vi "Goniometer2.vi"() -> ()   [LabVIEW 2024]
uses:
  F:/Desktop/Goniometer_Labview/ThorLabs.MotionControl.KCube.DCServoCLI.dll
  ThorLabs.MotionControl.KCube.DCServoCLI.dll
  F:/Desktop/Goniometer_Labview/Thorlabs.MotionControl.Controls.dll
  Thorlabs.MotionControl.Controls.dll
panel:
  in  "Boolean":bool
  out "이동거리":dbl[](array[numeric])
  out "Waveform Chart":dbl[](graph)
  out "XY Graph":cluster{dbl[], dbl[]}(graph)
  out "측정값":dbl[](array[numeric])
  out "error out":errorcluster {"code" format="%.0x"}
  in  "direction":i32(ring)=2 items=["Forward"=1, "Backward"=2]
  in  "목표위치":dbl
  in  "간격":dbl
  in  "Mode":u16(ring) items=["Current", "Power"]
  out "Current":dbl
  in  "Wavelength (0.0)":dbl=1064.0
  out "Power":dbl
  in  "Serial Number":string
  in  "KCubeDCServoControl":refnum<k24>(container)
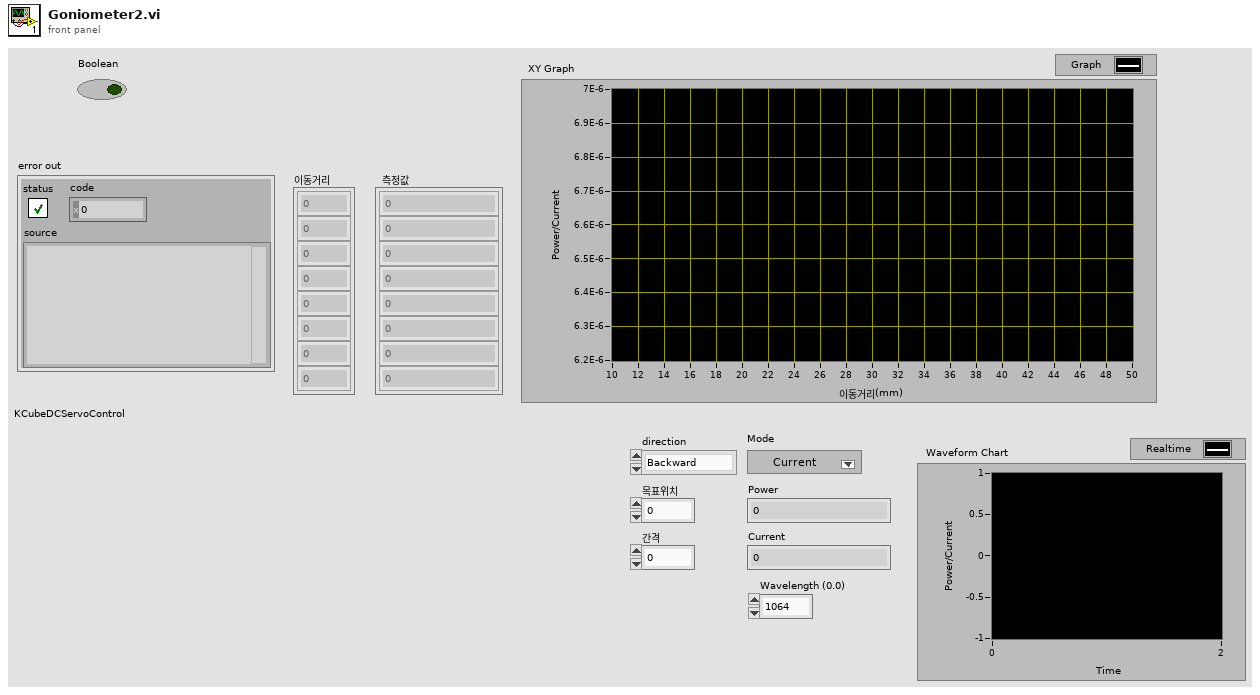
[diagram p1: front panel]
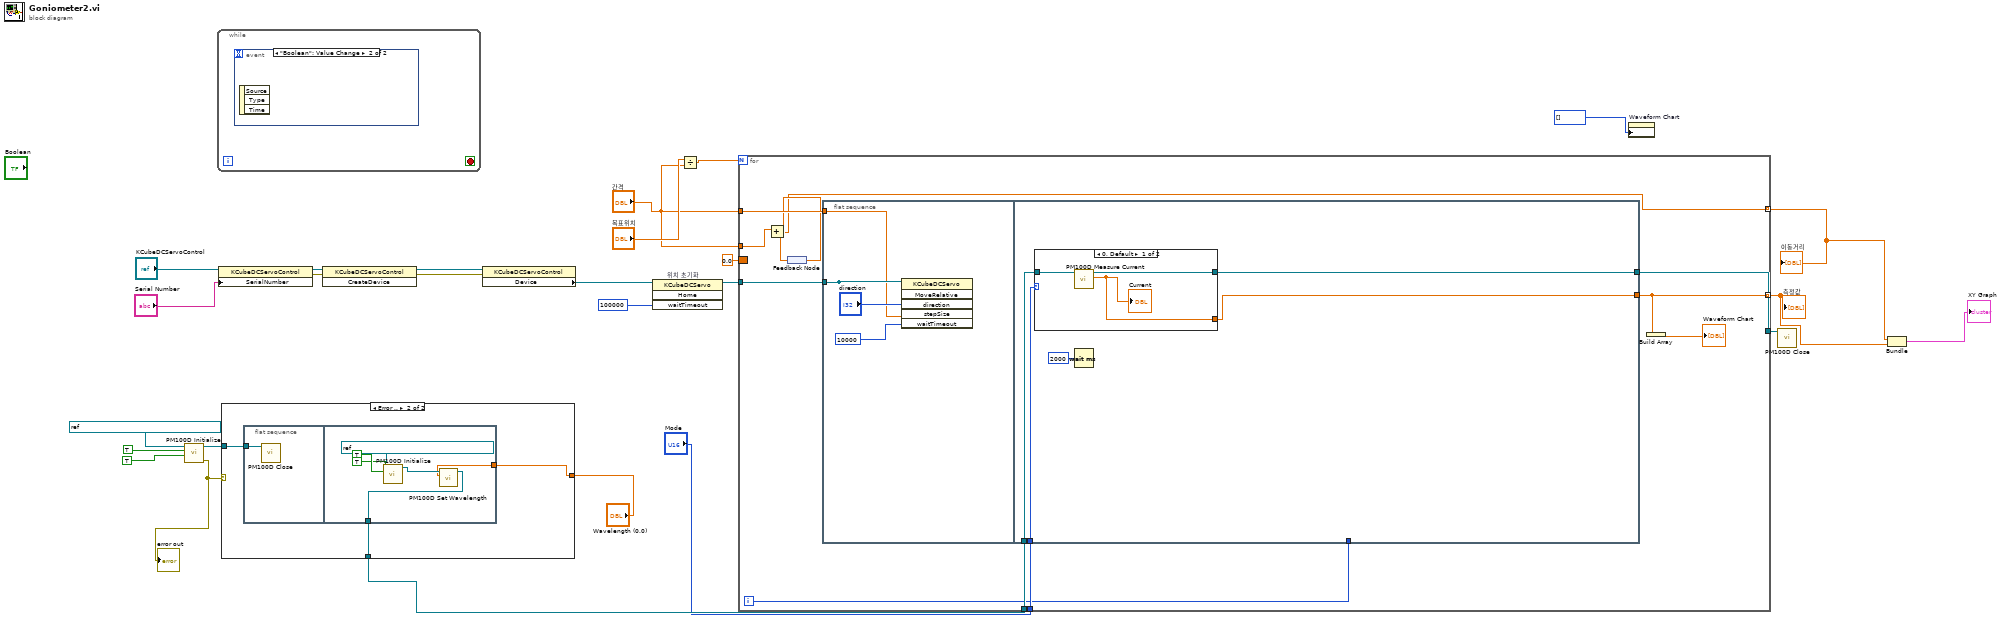
[diagram p0: block diagram]
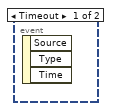
[diagram p2: hidden frame]
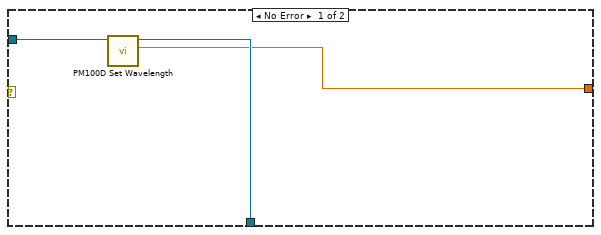
[diagram p3: hidden frame]
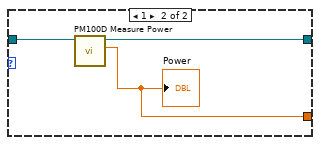
[diagram p4: hidden frame]
diagram:
  n1 = call <instrlib>:"PM100D Initialize.vi"("Reset Device (Reset Device)"=TRUE, "ID Query (Do Query)"=TRUE, "resource name"=refnum<visa-resource-name> "USB0::0x1313::0x8078::P0008024::INSTR") -> ("error out"=w8:errorcluster, "instrument handle out"=w17:refnum<visa-resource-name>)  [unwired: 7 in]
  "error out" <- w8
  n2 = while {
    stop <- _ stop-if-true
    n3 = event shown="[1] \"Boolean\": Value Change" {
      selector: _ -> [_ _]
      dyn-events: _ -> [_ _]
      timeout: _ -> [_ _]
      event Timeout {
        n4 = event-data() -> ()  [unwired: 1 in, 3 out]
      }
      event "Boolean": Value Change {
        n5 = event-data() -> ()  [unwired: 1 in, 3 out]
      }
    }
  }
  n6 = property class="KCubeDCServoControl"(reference="KCubeDCServoControl", "SerialNumber"="Serial Number") -> (reference out=w22:refnum<k24>, error out=w25:errorcluster)  [unwired: 1 in]
  n7 = case shown="Error .." w8 {
    tunnel: w17 -> [w29 w32]
    tunnel: [w28 w31] -> w14
    tunnel: "Wavelength (0.0)" -> [w27 w30]
    frame No Error {
      n8 = call <instrlib>:"PM100D Set Wavelength.vi"("Wavelength (0.0)"=w27, "instrument handle"=w29) -> ("instrument handle out"=w28:refnum<visa-resource-name>)  [unwired: 8 in, 1 out]
    }
    frame Error {
      n9 = flat-sequence {
        tunnel: w32 -> [w33]
        tunnel: [w35] -> w31
        tunnel: w30 -> [w34]
        frame #0 {
          n10 = call <instrlib>:"PM100D Close.vi"("instrument handle"=w33) -> ()  [unwired: 10 in, 1 out]
        }
        frame #1 {
          n11 = call <instrlib>:"PM100D Initialize.vi"("Reset Device (Reset Device)"=TRUE, "ID Query (Do Query)"=TRUE, "resource name"=refnum<visa-resource-name> "USB0::0x1313::0x8078::P0008024::INSTR") -> ("instrument handle out"=w36:refnum<visa-resource-name>)  [unwired: 7 in, 1 out]
          n12 = call <instrlib>:"PM100D Set Wavelength.vi"("Wavelength (0.0)"=w34, "instrument handle"=w36) -> ("instrument handle out"=w35:refnum<visa-resource-name>)  [unwired: 8 in, 1 out]
        }
      }
    }
  }
  n13 = invoke class="KCubeDCServoControl" method="CreateDevice"(reference=w22, error in=w25) -> (reference out=w23:refnum<k24>, error out=w26:errorcluster)  [unwired: 1 in, 1 out]
  n14 = property class="KCubeDCServoControl"(reference=w23, error in=w26) -> ("Device"=w11:refnum<k24>)  [unwired: 2 out]
  n15 = invoke on="위치 초기화" class="KCubeDCServo" method="Home"(reference=w11, "waitTimeout"=100000) -> (reference out=w10:refnum<k24>)  [unwired: 2 in, 3 out]
  n16 = Divide(x="목표위치", y="간격") -> (x/y=w16:dbl)
  n17 = for {
    N: w16 -> [_]
    tunnel: w10 -> [w50]
    tunnel: "Mode" -> [w49]
    tunnel: "간격" -> [w48]
    tunnel: w14 -> [w47]
    tunnel: [w46] -> w13
    tunnel: "간격" -> [w44]
    tunnel: [w42] -> w5 mode=indexing
    tunnel: [w40] -> w3 mode=indexing
    border: 0.0 -> [_]
    i -> [w45]
    n18 = feedback #1() -> (w43:dbl)
    n19 = Add(x=w44, y=w43) -> (x+y=w40:dbl)
    n20 = feedback-in #1(w40) -> ()
    n21 = flat-sequence {
      tunnel: w48 -> [w51]
      tunnel: w50 -> [w54]
      tunnel: [w54] -> _
      tunnel: w49 -> [w59]
      tunnel: w47 -> [w58]
      tunnel: [w57] -> w46
      tunnel: w45 -> [_]
      tunnel: [w55] -> w42
      frame #0 {
        n22 = invoke class="KCubeDCServo" method="MoveRelative"(reference=w54, "direction"="direction", "stepSize"=w51, "waitTimeout"=10000) -> ()  [unwired: 2 in, 6 out]
      }
      frame #1 {
        n23 = case shown="0, Default" w59 {
          tunnel: w58 -> [w61 w65]
          tunnel: [w62 w64] -> w57
          tunnel: [w60 w63] -> w55
          frame 0, Default {
            n24 = call <instrlib>:"PM100D Measure Current.vi"("instrument handle"=w61) -> ("Current"=w60:dbl, "instrument handle out"=w62:refnum<visa-resource-name>)  [unwired: 8 in, 1 out]
            "Current" <- w60
          }
          frame 1 {
            n25 = call <instrlib>:"PM100D Measure Power.vi"("instrument handle"=w65) -> ("Power"=w63:dbl, "instrument handle out"=w64:refnum<visa-resource-name>)  [unwired: 8 in, 1 out]
            "Power" <- w63
          }
        }
        n26 = Wait (ms)(milliseconds to wait=u32 2000) -> ()  [unwired: 1 out]
      }
    }
    n27 = Build Array(w42) -> (→"Waveform Chart":dbl[])
  }
  "측정값" <- w5
  "이동거리" <- w3
  n28 = property on="Waveform Chart" class="WFChart (strict)"("History Data"=i32[] []) -> ()  [unwired: 2 in, 2 out]
  n29 = call <instrlib>:"PM100D Close.vi"("instrument handle"=w13) -> ()  [unwired: 10 in, 1 out]
  n30 = Bundle(w3, w5) -> (→"XY Graph":cluster{dbl[], dbl[]})  [unwired: 1 in]
